vi "Carbide-Put-TargetPpDivider.vi"(8 "Error In":errorcluster, 11 "Value":i32) -> (0 "Error Out":errorcluster)   [LabVIEW 2014]
doc: "André Romero - 2021\nandretec@ifsc.usp.br\nIFSC - USP"
uses:
  Carbide-Global.vi
  <vilib>/httpClient/PUTBuffer.vi
  <vilib>/httpClient/LabVIEWHTTPClient.lvlib
panel:
  out "concatenated string":string
  out "body":string
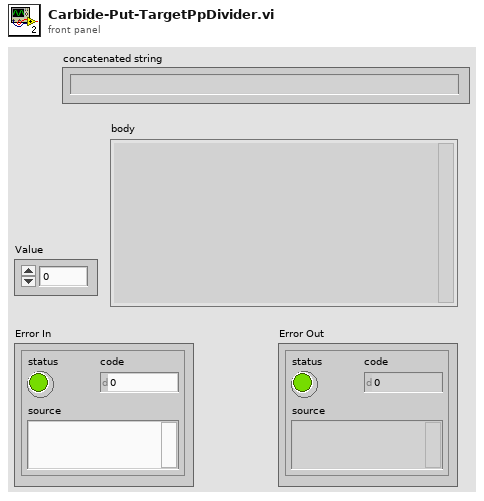
[diagram p1: front panel]
types:
  T1 = typedef "LabVIEWHTTPClient.lvlib/ClientHandle.ctl" = refnum<k1>
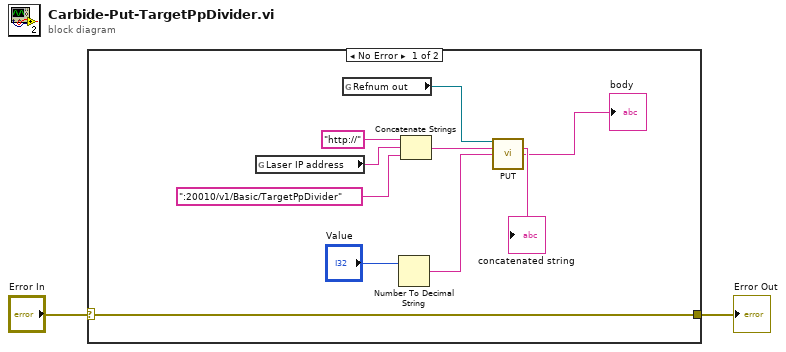
[diagram p0: block diagram]
diagram:
  n1 = case shown="No Error" "Error In" {
    selector: "Error In" -> [w6 w12]
    tunnel: [w6 w12] -> w1
    frame No Error {
      n2 = global read "Carbide-Global.vi" "Laser IP address"() -> (w8:string)
      n3 = global read "Carbide-Global.vi" "Refnum out"() -> (w11:T1)
      n4 = Number To Decimal String(number="Value") -> (decimal integer string=w4:string)  [unwired: 1 in]
      n5 = Concatenate Strings("http://" ("string"), w8, ":20010/v1/Basic/TargetPpDivider" ("string")) -> (w10:string)
      "concatenated string" <- w10
      n6 = call-poly <vilib>:"PUT.vi"("client handle"=w11, "url"=w10, "buffer"=w4) -> ("body"=→"body":string)  [unwired: 9 in, 3 out]
    }
    frame Error {
    }
  }
  "Error Out" <- w1
